vi "Scale Chart Axis.vi"(8 "V2":dbl, 10 "V1":dbl, 11 "Chart":refnum<vi>) -> (3 "Chart":cluster{"Viscosity":dbl, "Temperature":dbl})   [LabVIEW 2019]
uses:
  <vilib>/ptbypt/NI_PtbyPt.lvlib
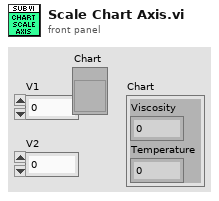
[diagram p1: front panel]
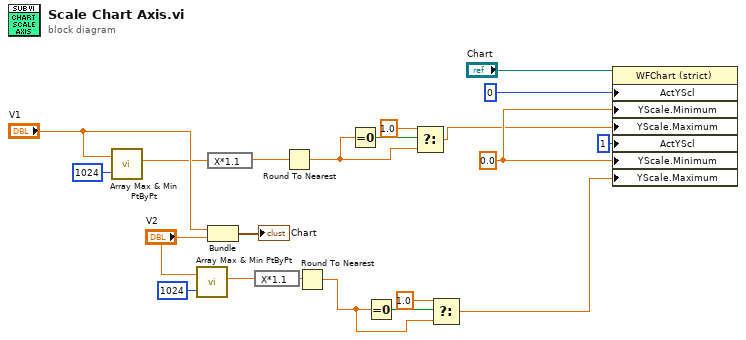
[diagram p0: block diagram]
diagram:
  w20 = 0.0 ("X Scale.Range:Start")
  n1 = call <vilib>:"Array Max & Min PtByPt.vi"("input data point"="V1", "sample length"=1024) -> ("max value"=w12:dbl)  [unwired: 1 in, 4 out]
  n2 = call <vilib>:"Array Max & Min PtByPt.vi"("input data point"="V2", "sample length"=1024) -> ("max value"=w10:dbl)  [unwired: 1 in, 4 out]
  n3 = expression code="X*1.1"(w12) -> (w11:dbl)
  n4 = Bundle("V1"="V1", "V2"="V2") -> (→"Chart":cluster{"V1":dbl, "V2":dbl})  [unwired: 1 in]
  n5 = expression code="X*1.1"(w10) -> (w9:dbl)
  n6 = Round To Nearest(number=w11) -> (nearest integer value=w6:dbl)
  n7 = Round To Nearest(number=w9) -> (nearest integer value=w2:dbl)
  n8 = Equal To 0?(x=w6) -> (x = 0?=w8:bool)
  n9 = Equal To 0?(x=w2) -> (x = 0?=w3:bool)
  n10 = Select(t=1.0, s=w8, f=w6) -> (s? t:f=w5:dbl)
  n11 = Select(t=1.0, s=w3, f=w2) -> (s? t:f=w1:dbl)
  n12 = property on="Property Node" class="WFChart (strict)"(reference="Chart", "ActYScl"=u32 0 ("Active Plot"), "YScale.Minimum"=w20, "YScale.Maximum"=w5, "ActYScl"=1 ("Active Y Scale"), "YScale.Minimum"=w20, "YScale.Maximum"=w1) -> ()  [unwired: 1 in, 2 out]
